vi "Untitled 3.vi"() -> ()   [LabVIEW 2016, in "Example Source.lvlib" / "Example Source.lvclass"]
uses:
  Examples/Example Source/Example Source/Example Source.lvclass
  Examples/Example Source/Example Events/Double Array Event.lvclass
  C:/Projects/Shared Libraries/Event Actors/Event/Event.lvclass
  Event/Event.lvclass/Event.ctl
  Event/Event.lvclass
panel:
  out "Event ID":string
  out "data string 3":string
  out "data string 2":string
  out "data string":string
  in  "Example Source.lvlib:Double Array Event.lvclass":refnum<class "Double Array Event.lvclass">
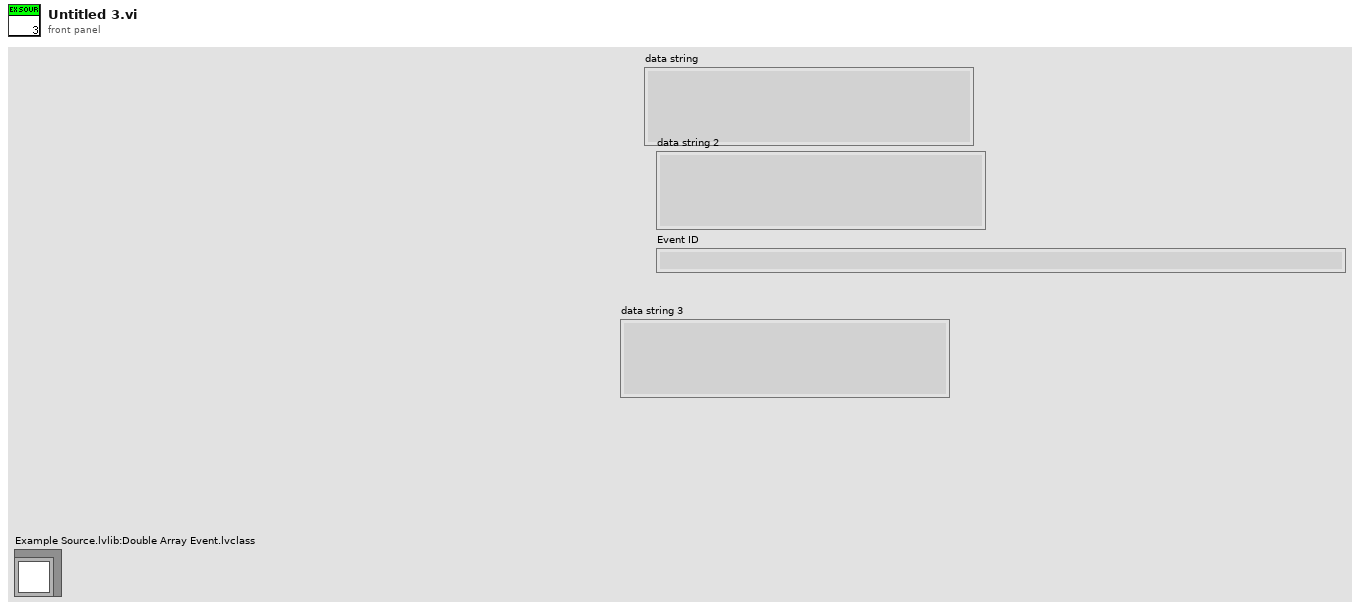
[diagram p1: front panel]
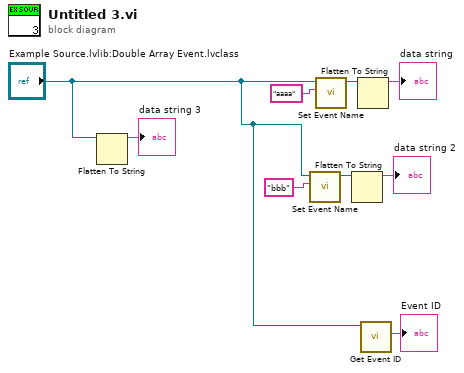
[diagram p0: block diagram]
diagram:
  n1 = Flatten To String(anything="Example Source.lvlib:Double Array Event.lvclass") -> (data string=→"data string 3":string)  [unwired: 3 in, 2 out]
  n2 = call "Set Event Name.vi"("Name (Generic)"="bbb", "Event In"="Example Source.lvlib:Double Array Event.lvclass") -> ("Event Out"=w4:refnum<class "Double Array Event.lvclass">)  [unwired: 9 in]
  n3 = call "Set Event Name.vi"("Name (Generic)"="aaaa", "Event In"="Example Source.lvlib:Double Array Event.lvclass") -> ("Event Out"=w7:refnum<class "Double Array Event.lvclass">)  [unwired: 9 in]
  n4 = Flatten To String(anything=w4) -> (data string=→"data string 2":string)  [unwired: 3 in, 2 out]
  n5 = Flatten To String(anything=w7) -> (data string=→"data string":string)  [unwired: 3 in, 2 out]
  n6 = call-dynamic "Get Event ID.vi"("Event in"="Example Source.lvlib:Double Array Event.lvclass") -> ("Event ID"=→"Event ID":string)  [unwired: 8 in, 2 out]
